vi "WriteCalibrationToFile (SubVI).vi"(0 "Stave ID":string, 1 "User notes":string, 2 "CameraWD":dbl format="%#_13g", 3 "um/Pixel":dbl format="%#_13g", 4 "Angle":dbl format="%#_13g", 5 "Stave Origin":dbl[](array[numeric]), 7 "error in (no error)":errorcluster, 8 "Calibration file path":path, 10 "Write to file":bool=TRUE, 17 "Stave Configuration File":path, 18 "StaveOrientationString":string, 19 "ToolingPinOrientationString":string) -> (13 "error out":errorcluster)   [LabVIEW 2016]
uses:
  <vilib>/Utility/config.llb/Write Key (String).vi
  <vilib>/Utility/config.llb/Write Key (Double).vi
  <vilib>/Utility/config.llb/NI_LVConfig.lvlib
panel:
  # "General"
  # "Camera Calibration"
  # "Stave basis calibration"
  # "(Date and time recorded)"
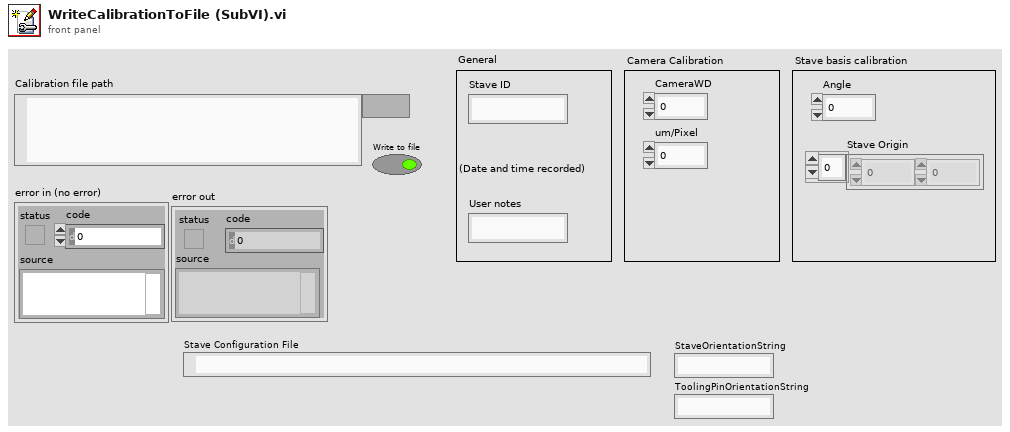
[diagram p1: front panel]
types:
  T1 = typedef "NI_LVConfig.lvlib/Config Data RefNum.ctl" = refnum<k1>
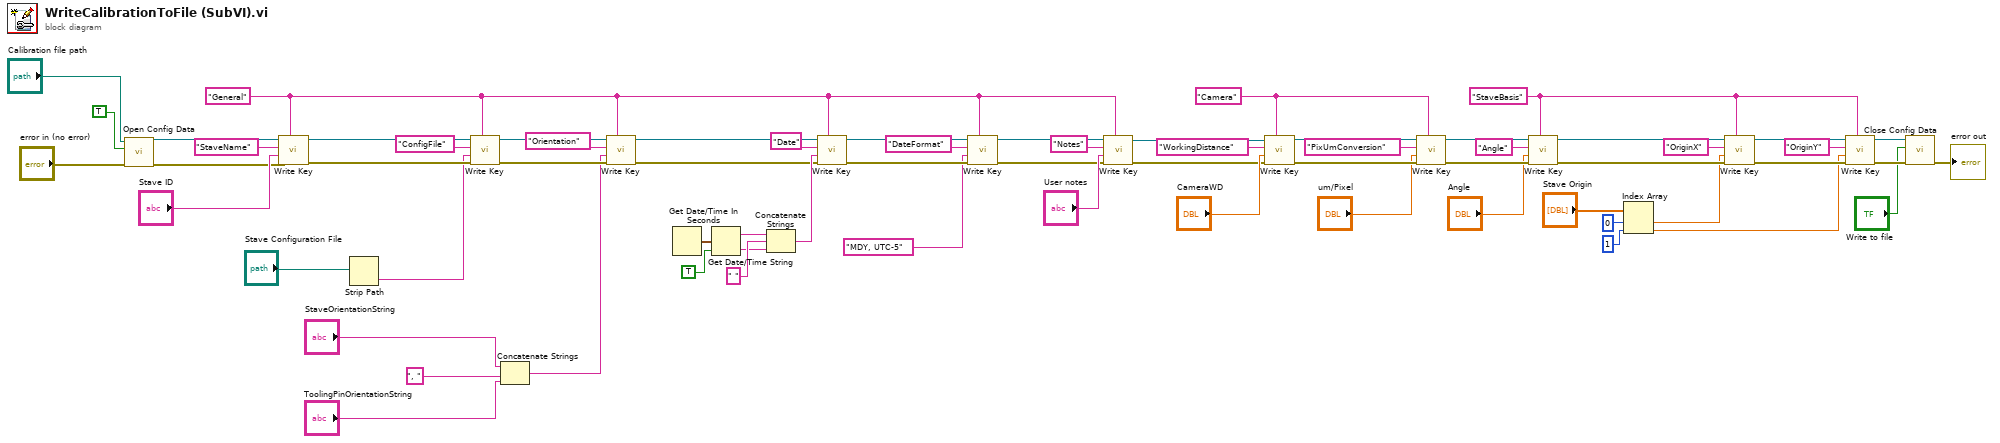
[diagram p0: block diagram]
diagram:
  w30 = "StaveBasis" ("section")
  w41 = "Camera" ("section")
  w1 = "General" ("section")
  n1 = call <vilib>:"Open Config Data.vi"("error in (no error)"="error in (no error)", "create file if necessary (T)"=TRUE, "configuration file path"="Calibration file path") -> ("error out"=w60:errorcluster, "refnum"=w63:T1)  [unwired: 6 in, 1 out]
  n2 = call-poly <vilib>:"Write Key.vi"("section"=w1, "error in (no error)"=w60, "value"="Stave ID", "key"="StaveName", "refnum"=w63) -> ("error out"=w21:errorcluster, "refnum out"=w22:T1)  [unwired: 4 in, 1 out]
  n3 = Strip Path(path="Stave Configuration File") -> (name=w3:string)  [unwired: 1 out]
  n4 = call-poly <vilib>:"Write Key.vi"("section"=w1, "error in (no error)"=w21, "value"=w3, "key"="ConfigFile", "refnum"=w22) -> ("error out"=w18:errorcluster, "refnum out"=w19:T1)  [unwired: 4 in, 1 out]
  n5 = Concatenate Strings("StaveOrientationString", ", ", "ToolingPinOrientationString") -> (w5:string)
  n6 = call-poly <vilib>:"Write Key.vi"("section"=w1, "error in (no error)"=w18, "value"=w5, "key"="Orientation", "refnum"=w19) -> ("error out"=w10:errorcluster, "refnum out"=w11:T1)  [unwired: 4 in, 1 out]
  n7 = Get Date/Time In Seconds() -> (seconds since 1Jan1904=w57:timestamp)
  n8 = Get Date/Time String(seconds (now)=w57, want seconds? (F)=TRUE) -> (date string=w55:string, time string=w54:string)  [unwired: 1 in]
  n9 = Concatenate Strings(w55, " " ("string"), w54) -> (w53:string)
  n10 = call-poly <vilib>:"Write Key.vi"("section"=w1, "error in (no error)"=w10, "value"=w53, "key"="Date", "refnum"=w11) -> ("error out"=w13:errorcluster, "refnum out"=w16:T1)  [unwired: 4 in, 1 out]
  n11 = call-poly <vilib>:"Write Key.vi"("section"=w1, "error in (no error)"=w13, "value"="MDY, UTC-5" ("key"), "key"="DateFormat", "refnum"=w16) -> ("error out"=w14:errorcluster, "refnum out"=w15:T1)  [unwired: 4 in, 1 out]
  n12 = call-poly <vilib>:"Write Key.vi"("section"=w1, "error in (no error)"=w14, "value"="User notes", "key"="Notes", "refnum"=w15) -> ("error out"=w43:errorcluster, "refnum out"=w42:T1)  [unwired: 4 in, 1 out]
  n13 = call-poly <vilib>:"Write Key.vi"("section"=w41, "error in (no error)"=w43, "value"="CameraWD", "key"="WorkingDistance", "refnum"=w42) -> ("error out"=w51:errorcluster, "refnum out"=w46:T1)  [unwired: 4 in, 1 out]
  n14 = call-poly <vilib>:"Write Key.vi"("section"=w41, "error in (no error)"=w51, "value"="um/Pixel", "key"="PixUmConversion", "refnum"=w46) -> ("error out"=w50:errorcluster, "refnum out"=w49:T1)  [unwired: 4 in, 1 out]
  n15 = call-poly <vilib>:"Write Key.vi"("section"=w30, "error in (no error)"=w50, "value"="Angle", "key"="Angle", "refnum"=w49) -> ("error out"=w37:errorcluster, "refnum out"=w34:T1)  [unwired: 4 in, 1 out]
  n16 = Index Array(array="Stave Origin", index #1=0 ("index"), index #2=1 ("index")) -> (element #1=w25:dbl, element #2=w24:dbl)
  n17 = call-poly <vilib>:"Write Key.vi"("section"=w30, "error in (no error)"=w37, "value"=w25, "key"="OriginX", "refnum"=w34) -> ("error out"=w36:errorcluster, "refnum out"=w35:T1)  [unwired: 4 in, 1 out]
  n18 = call-poly <vilib>:"Write Key.vi"("section"=w30, "error in (no error)"=w36, "value"=w24, "key"="OriginY", "refnum"=w35) -> ("error out"=w32:errorcluster, "refnum out"=w33:T1)  [unwired: 4 in, 1 out]
  n19 = call <vilib>:"Close Config Data.vi"("error in (no error)"=w32, "write file if changed (T)"="Write to file", "refnum"=w33) -> ("error out"=→"error out":errorcluster)  [unwired: 7 in, 1 out]
